vi "getInfo.vi"(6 "LabVIEW Web Service Request":refnum<class "Web Request.lvclass"> caption="LabVIEW Web服务请求") -> (0 "aveData":dbl, 1 "minData":dbl, 2 "maxData":dbl, 3 "realtimeData":dbl)   [LabVIEW 2014]
doc: "This example shows how to configure a measurement and take a single reading."
uses:
  <vilib>/wsapi/Web Request.lvclass
  Fluke 884X Series/Public/Data/Read (Single Point).vi
  Fluke 884X Series/Fluke 884X Series.lvlib
panel:
  in  "测试项目":u16(ring)=4 items=["DC Voltage", "AC Voltage", "2 - Wire Resistance", "4 - Wire Resistance", "DC Current", "AC Current", "Frequency", "Period", "Continuity", "Diode Checking", "Temperature", "Capacitance"]
  out "电压/电流":dbl[](graph)
  in  "串口":refnum<visa-resource-name>
  # "FLUKE 8846A台式万用表静电流采集V2.0"
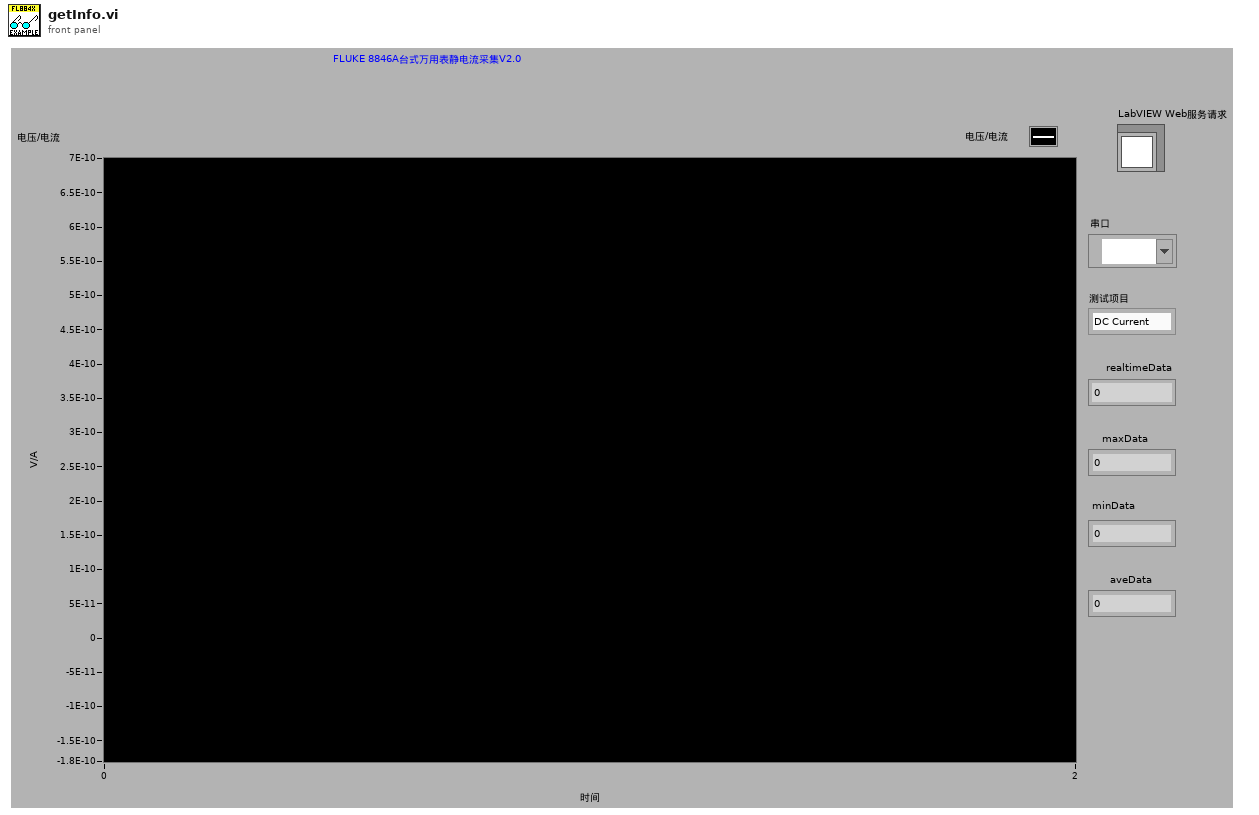
[diagram p1: front panel]
types:
  T1 = cluster{"Baud Rate":u32, "Parity":u16, "Data Bits":u16, "Stop Bits":u16, "Flow Control":u16}
  T2 = enum16{"None", "Min/Max", "Null", "dB", "dBm", "Limit"}
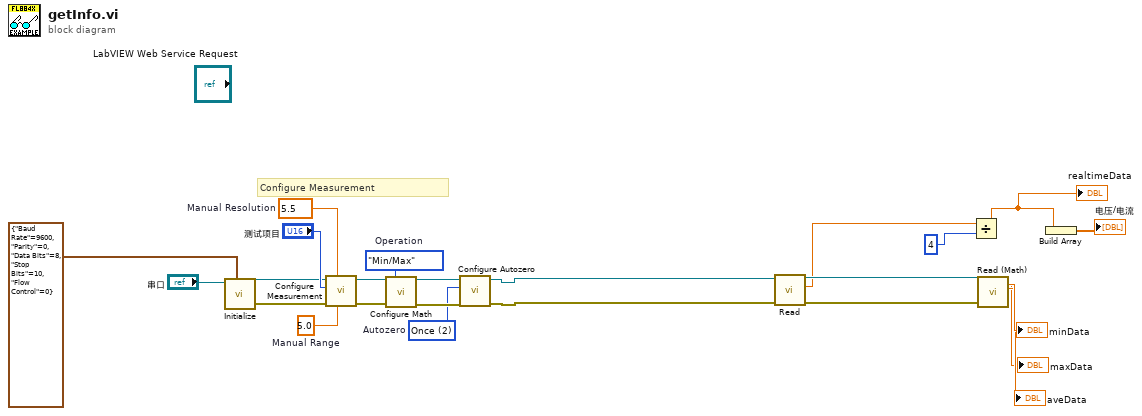
[diagram p0: block diagram]
diagram:
  w15 = 5.0  # Manual Range
  w16 = 5.5 items=["4.5"=4.5, "5.5"=5.5, "6.5"=6.5]  # Manual Resolution
  w17 = u16 2 items=["On", "Off", "Once"]  # Autozero
  w18 = T2."Min/Max"  # Operation
  # "Configure Measurement"
  n1 = call "Initialize.vi"("Serial Configuration"=T1 {"Baud Rate"=9600, "Parity"=0, "Data Bits"=8, "Stop Bits"=10, "Flow Control"=0}, "VISA resource name"="串口") -> ("error out"=w13:errorcluster, "VISA resource name out"=w14:refnum<visa-resource-name>)  [unwired: 8 in]
  n2 = call "Configure Measurement.vi"("Manual Range (1.0)"=w15, "Manual Resolution (5.5 Digits)"=w16, "error in (no error)"=w13, "Function (0: DC Voltage)"="测试项目", "VISA resource name"=w14) -> ("error out"=w22:errorcluster, "VISA resource name out"=w23:refnum<visa-resource-name>)  [unwired: 5 in]
  n3 = call "Configure Math.vi"("VISA resource name"=w23, "Operation (0:None)"=w18, "error in (no error)"=w22) -> ("VISA resource name out"=w21:refnum<visa-resource-name>, "error out"=w20:errorcluster)  [unwired: 11 in]
  n4 = call "Configure Autozero.vi"("error in (no error)"=w20, "Autozero  (0: On)"=w17, "VISA resource name"=w21) -> ("error out"=w11:errorcluster, "VISA resource name out"=w12:refnum<visa-resource-name>)  [unwired: 7 in]
  n5 = call-poly "Read.vi"("error in (no error)"=w11, "VISA resource name"=w12) -> ("error out"=w4:errorcluster, "Measurement"=w3:dbl, "VISA resource name out"=w5:refnum<visa-resource-name>)  [unwired: 7 in]
  n6 = Divide(x=w3, y=4) -> (x/y=w1:dbl)
  "realtimeData" <- w1
  n7 = call "Read (Math).vi"("error in (no error)"=w4, "VISA resource name"=w5) -> ("Average"=→"aveData":dbl, "Minimum"=→"minData":dbl, "Maximum"=→"maxData":dbl)  [unwired: 4 in, 3 out]
  n8 = Build Array(w1) -> (→"电压/电流":dbl[])
